vi "PH_gentec_P-Link.set Trigger Polarity.vi"(0 "i ref in":refnum<vi>, 2 "VISA resource in":refnum<visa-resource-name>, 5 "error in":errorcluster) -> (11 "Timeout":bool, 13 "Data read":string[](array[string]), 14 "i ref out":refnum<vi>, 16 "VISA resource out":refnum<visa-resource-name>, 17 "Error":bool, 18 "Failure":bool, 19 "error out":errorcluster)   [LabVIEW 2014, in "PH_gentec_P-Link.lvlib"]
doc: "This VI writes wanted Settings to the Device and checks the result."
uses:
  PH_gentec_P-Link.lvlib
  instr.lib/Gentec-M-Link/gentec-M-Link - Driver.lvlib
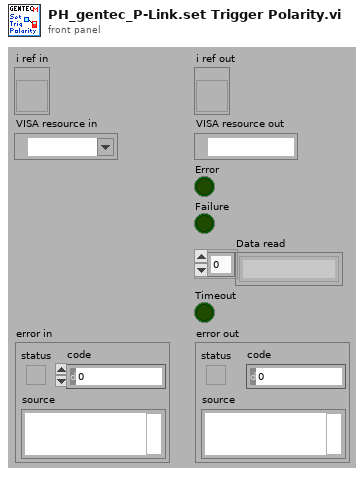
[diagram p1: front panel]
types:
  T1 = typedef "PH_gentec_P-Link.lvlib/PH_gentec_P-Link.i attribute.ctl" = cluster{"GUI References":cluster{"Wanted Head Settings":refnum<vi>, "Current Head Settings":refnum<vi>, "Set Auto Range":refnum<vi>, "Trigger Polarity":refnum<vi>, "Trigger Source":refnum<vi>, "Waveform Averages":refnum<vi>, "Continuous":refnum<vi>, "get one Value":refnum<vi>}, "Wanted Head Settings":T2, "Current Head Settings":T2}
  T2 = typedef "PH_gentec_P-Link.lvlib/PH_gentec_P-Link.Head Settings.ctl" = cluster{"Measurement Mode":T3, "Enable Anticipation":bool, "Set Auto Range":bool, "Block Signal":bool, "Set Head Attenuator":bool, "Enable SSE":bool, "Trigger Polarity":T4, "Trigger Source":T5, "Waveform Averages":T6, "Set Zero":i32, "Current Measurement":i32, "Start Data Flow":bool}
  T3 = typedef "gentec-M-Link - Driver.lvlib/gentec-M-Link.Measurement Mode.ctl" = u16
  T4 = typedef "gentec-M-Link - Driver.lvlib/gentec-M-Link.Trigger Polarity.ctl" = u16
  T5 = typedef "gentec-M-Link - Driver.lvlib/gentec-M-Link.Trigger Source.ctl" = u16
  T6 = typedef "gentec-M-Link - Driver.lvlib/gentec-M-Link.Waveform Averages.ctl" = u16
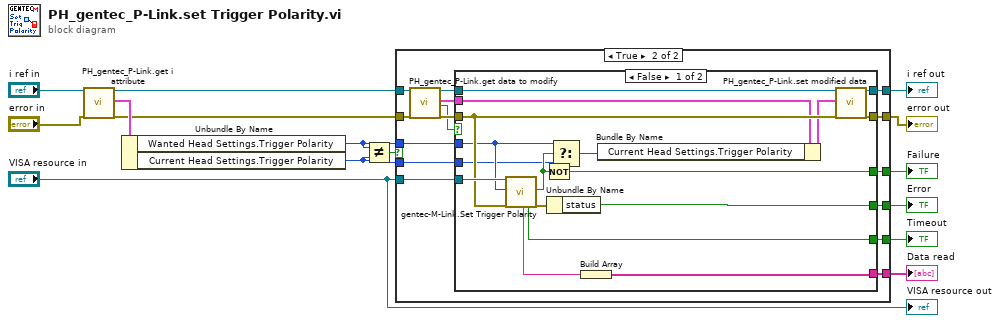
[diagram p0: block diagram]
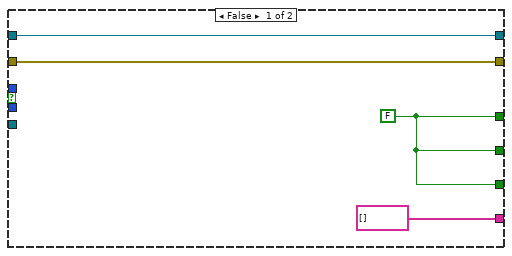
[diagram p2: hidden frame]
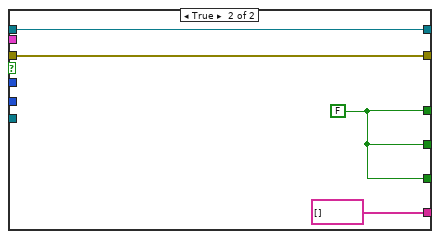
[diagram p3: hidden frame]
diagram:
  n1 = call "PH_gentec_P-Link.get i attribute.vi"("i ref in"="i ref in", "error in (no error)"="error in") -> ("i ref out"=w9:refnum<vi>, "i attribute"=w12:T1, "error out"=w11:errorcluster)  [unwired: 15 in]
  n2 = Unbundle By Name(w12) -> ("Wanted Head Settings.Trigger Polarity"=w13:T4, "Current Head Settings.Trigger Polarity"=w1:T4)
  n3 = Not Equal?(x=w13, y=w1) -> (x != y?=w2:bool)
  n4 = case shown="True" w2 {
    tunnel: [w16 w34] -> w15
    tunnel: [w17 w33] -> w14
    tunnel: w13 -> [_ w32]
    tunnel: w11 -> [w16 w27]
    tunnel: w9 -> [w17 w26]
    tunnel: "VISA resource in" -> [_ w25]
    tunnel: [w19 w24] -> w6
    tunnel: [w19 w23] -> w5
    tunnel: [w19 w22] -> w4
    tunnel: [string[] [] w21] -> w3
    tunnel: w1 -> [_ w20]
    frame False {
      w19 = FALSE
    }
    frame True {
      n5 = call "PH_gentec_P-Link.get data to modify.vi"("i ref in"=w26, "error in (no error)"=w27) -> ("i ref out"=w30:refnum<vi>, "i attribute"=w29:T1, "timed out"=w28:bool, "error out"=w31:errorcluster)  [unwired: 14 in]
      n6 = case shown="False" w28 {
        tunnel: w25 -> [w50 _]
        tunnel: [w47 w55] -> w33
        tunnel: [w46 w54] -> w34
        tunnel: w31 -> [w49 w54]
        tunnel: w30 -> [w51 w55]
        tunnel: w29 -> [w48 _]
        tunnel: w32 -> [w39 _]
        tunnel: [w44 w53] -> w24
        tunnel: [w37 w53] -> w23
        tunnel: [w43 w53] -> w22
        tunnel: [w42 string[] []] -> w21
        tunnel: w20 -> [w35 _]
        frame False {
          n7 = call "gentec-M-Link.Set Trigger Polarity.vi"("VISA resource In"=w50, "Trigger Polarity"=w39, "error in (no error)"=w49) -> ("Data Read"=w41:string, "Read Timeout"=w43:bool, "Success"=w38:bool, "error out"=w36:errorcluster)  [unwired: 12 in, 1 out]
          n8 = Not(x=w38) -> (.not. x?=w37:bool)
          n9 = Unbundle By Name(w36) -> ("status"=w44:bool)
          n10 = Select(t=w39, s=w38, f=w35) -> (s? t:f=w40:T4)
          n11 = Build Array(w41) -> (w42:string[])
          n12 = Bundle By Name(cluster=w48, "Current Head Settings.Trigger Polarity"=w40) -> (w45:T1)
          n13 = call "PH_gentec_P-Link.set modified data.vi"("i ref in"=w51, "i attribute"=w45, "error in (no error)"=w49) -> ("i ref out"=w47:refnum<vi>, "error out"=w46:errorcluster)  [unwired: 15 in]
        }
        frame True {
          w53 = FALSE
        }
      }
    }
  }
  "error out" <- w15
  "i ref out" <- w14
  "Error" <- w6
  "Failure" <- w5
  "Timeout" <- w4
  "Data read" <- w3
  "VISA resource out" <- "VISA resource in"
